vi "load tags from CVT3.vi"(10 "path":path, 11 "engine ref":refnum<data-value>) -> (2 "load attempted":bool)   [LabVIEW 2013, in "PL Framework Configuration Tool.lvlib" / "EngineTags.lvclass"]
uses:
  EngineTags.lvclass
  Engine Parent/Engine Parent Editor Node.lvclass
  <vilib>/NI/Module Execution Interface/Engine Configuration/engine configuration.lvclass
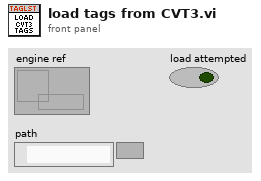
[diagram p1: front panel]
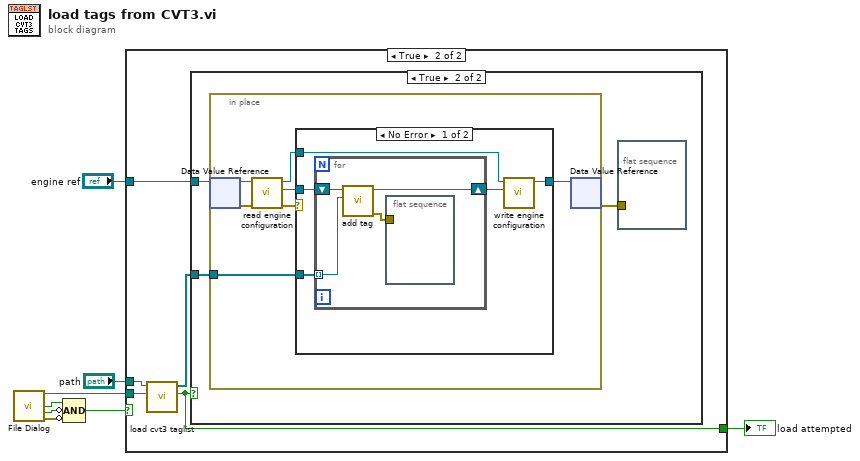
[diagram p0: block diagram]
diagram:
  n1 = call "File Dialog"() -> ("selected path"=w5:path, "exists"=w4:bool, "cancelled"=w3:bool, "error out"=w2:errorcluster)  [unwired: 12 in]
  n2 = Compound Arithmetic op=AND(w4, invert w3, invert w2) -> (w6:bool)
  n3 = case shown="True" w6 {
    tunnel: w5 -> [_ w11]
    tunnel: "path" -> [_ w13]
    tunnel: [_ w10] -> w8
    tunnel: "engine ref" -> [_ w9]
    frame False {
    }
    frame True {
      n4 = call "load cvt3 taglist.vi"("cfg file path"=w11, "vi path"=w13) -> ("ok?"=w10:bool, "tags"=w12:refnum<class "tag descriptor.lvclass">[])  [unwired: 8 in]
      n5 = case shown="True" w10 {
        tunnel: w12 -> [_ w14]
        tunnel: w9 -> [_ w15]
        frame False {
        }
        frame True {
          n6 = in-place {
            in-place-border: w14 -> [w23]
            n7 = in-place-dvr #1(w15) -> (w21:refnum<class "Engine Parent Editor Node.lvclass">, w22:errorcluster)
            n8 = call "read engine configuration.vi"("error in"=w22, "Engine Parent Editor Node in"=w21) -> ("error out"=w18:errorcluster, "engine configuration"=w17:refnum<class "engine configuration.lvclass">, "Engine Parent Editor Node out"=w20:refnum<class "Engine Parent Editor Node.lvclass">)  [unwired: 7 in]
            n9 = case shown="No Error" w18 {
              tunnel: w23 -> [w28 _]
              tunnel: w20 -> [w26 w33]
              tunnel: [w25 w33] -> w19
              tunnel: w17 -> [w24 _]
              frame No Error {
                n10 = for {
                  shift-right: [w32] -> w27
                  shift-left: w24 -> [w31]
                  tunnel: w28 -> [w30] mode=indexing
                  n11 = call <vilib>:"add tag.vi"("tag descriptor"=w30, "engine configuration in"=w31) -> ("error out"=w29:errorcluster, "engine configuration out"=w32:refnum<class "engine configuration.lvclass">)  [unwired: 8 in]
                  n12 = flat-sequence {
                    tunnel: w29 -> [_]
                    frame #0 {
                    }
                  }
                }
                n13 = call "write engine configuration.vi"("engine configuration"=w27, "Engine Parent Editor Node in"=w26) -> ("Engine Parent Editor Node out"=w25:refnum<class "Engine Parent Editor Node.lvclass">)  [unwired: 8 in, 1 out]
              }
              frame Error {
              }
            }
            n14 = in-place-dvr #1(w19) -> (w16:errorcluster)  [unwired: 1 out]
          }
          n15 = flat-sequence {
            tunnel: w16 -> [_]
            frame #0 {
            }
          }
        }
      }
    }
  }
  "load attempted" <- w8
